vi "ReadTektronixISF.vi"(5 "Length":i32, 7 "Start":i64, 8 "error in (no error)":errorcluster, 11 "Path":path) -> (0 "error out":errorcluster, 2 "dt":dbl=2e-10 format="%#_2e", 3 "Data":dbl[](array[numeric]), 4 "Total number of points":u64)   [LabVIEW 2021]
doc: "Reads an array of data from a byte stream binary file. By default, the VI is configured to read 8-byte (data type DBL) Little Endian Data. To modify the way sample data is read from the file, change the Byte Order and the value of the Byte Size (normal sizes are 1, 2, 4, or 8). If you change the byte size, also change the representation of the Data Type constant (default is DBL) to coincide with the byte size (1 = I8, 2 = I16, 4 = I32, 8 = DBL). Use the Write Binary File VI in this LLB to create the file.\n\nThis example was built using LabVIEW 8.0"
panel:
  out "Y Multiplier":dbl=3.125e-06
  out "Header Information":string=":WFMPRE:NR_PT 1000000;:WFMPRE:BYT_NR 2;BIT_NR 16;ENCDG BIN;BN_FMT RI;BYT_OR MSB;WFID \"Ch1, DC coupling, 20.00mV/div, 20.00us/div, 1000000 points, Sample mode\";NR_PT 1000000;PT_FMT Y;XUNIT \"s\";XINCR 200.0000E-12;XZERO -100.0000E-6;PT_OFF 0;YUNIT \"V\";YMULT 3.1250E-6;YOFF 0.0000;YZERO 0.0000;VSCALE 20.0000E-3;HSCALE 20.0000E-6;VPOS 0.0000;VOFFSET 0.0000;HDELAY 0.0000;:CURVE #72000000&\u0000#\u0000\u001f"
  out "output 1":i32=375
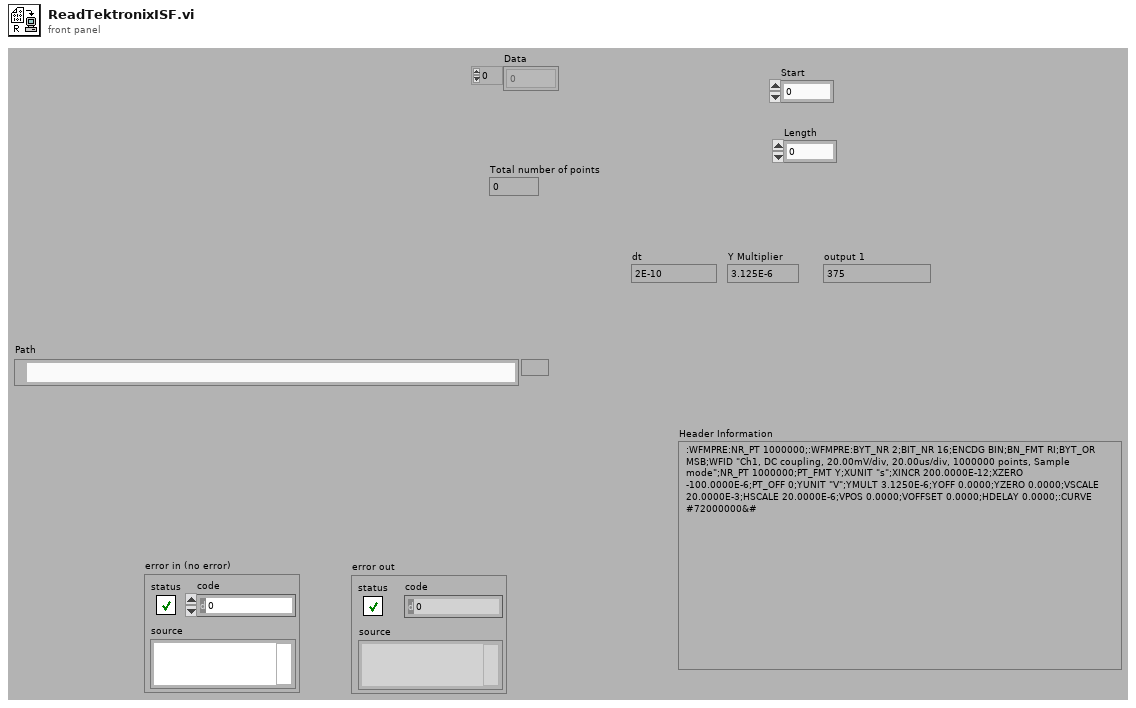
[diagram p1: front panel]
types:
  T1 = enum16{"open", "replace", "create", "open or create", "replace or create", "replace or create with confirmation"}
  T2 = enum16{"deny read/write", "deny write-only", "deny none"}
  T3 = enum16{"big-endian, network order", "native, host order", "little-endian"}
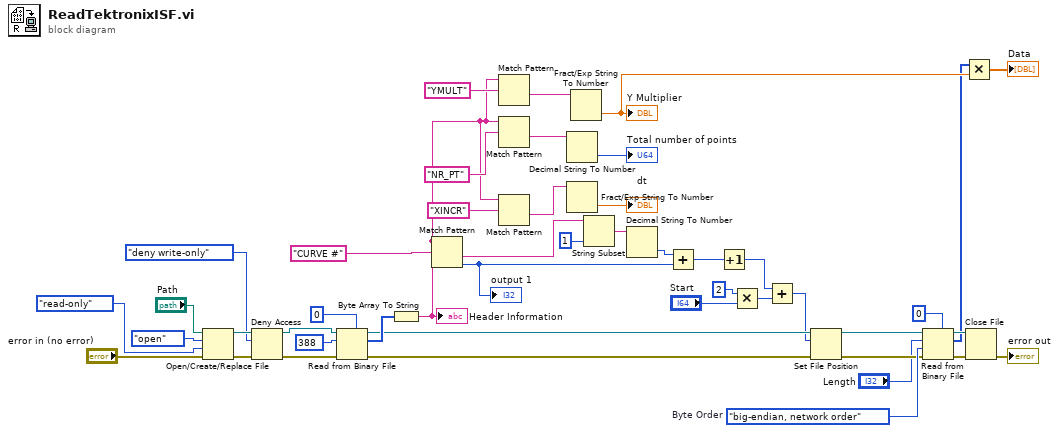
[diagram p0: block diagram]
diagram:
  w45 = T3."big-endian, network order"  # Byte Order
  n1 = Open/Create/Replace File(file path (use dialog)="Path", error in="error in (no error)", operation (0:open)=T1."open", access (0:read/write)=enum16{"read/write", "read-only", "write-only"}."read-only") -> (refnum out=w43:refnum<file>, error out=w44:errorcluster)  [unwired: 3 out]
  n2 = Deny Access(4:w44, 6:T2."deny write-only" ("deny mode (0:deny read/write)"), 7:w43) -> (0:w30:errorcluster, 3:w26:refnum<file>)
  n3 = Read from Binary File(5:u8 0, 8:w30, 10:388 ("count"), 11:w26) -> (0:w21:errorcluster, 2:w28:u8[], 3:w20:refnum<file>)  [unwired: 3 out]
  n4 = Byte Array To String(unsigned byte array=w28) -> (string=w27:string)
  "Header Information" <- w27
  n5 = Match Pattern(string=w27, regular expression="CURVE #") -> (after substring=w11:string, offset past match=w7:i32)  [unwired: 3 out]
  "output 1" <- w7
  n6 = Match Pattern(string=w27, regular expression="YMULT") -> (after substring=w3:string)  [unwired: 4 out]
  n7 = Match Pattern(string=w27, regular expression="NR_PT") -> (after substring=w1:string)  [unwired: 4 out]
  n8 = Match Pattern(string=w27, regular expression="XINCR") -> (after substring=w2:string)  [unwired: 4 out]
  n9 = Decimal String To Number(string=w1) -> (number=→"Total number of points":i32)  [unwired: 3 out]
  n10 = Fract/Exp String To Number(string=w2) -> (number=→"dt":dbl)  [unwired: 4 out]
  n11 = Fract/Exp String To Number(string=w3) -> (number=w37:dbl)  [unwired: 4 out]
  "Y Multiplier" <- w37
  n12 = String Subset(string=w11, length (rest)=1 ("length (rest)")) -> (substring=w8:string)  [unwired: 1 out]
  n13 = Decimal String To Number(string=w8) -> (number=w9:i32)  [unwired: 3 out]
  n14 = Add(x=w9, y=w7) -> (x+y=w6:i32)
  n15 = Increment(x=w6) -> (x+1=w5:i32)
  n16 = Multiply(x=i64 2, y="Start") -> (x*y=w23:i64)
  n17 = Add(x=w5, y=w23) -> (x+y=w19:i64)
  n18 = Set File Position(offset (in bytes) (0)=w19, refnum=w20, error in=w21) -> (refnum out=w17:refnum<file>, error out=w18:errorcluster)  [unwired: 1 out]
  n19 = Read from Binary File(5:i16 0, 8:w18, 9:w45, 10:"Length", 11:w17) -> (0:w15:errorcluster, 2:w13:i16[], 3:w16:refnum<file>)  [unwired: 2 out]
  n20 = Multiply(x=w13, y=w37) -> (x*y=→"Data":dbl[])
  n21 = Close File(refnum=w16, error in=w15) -> (error out=→"error out":errorcluster)  [unwired: 1 out]
